vi "Reentrant SubVI.vi"(11 "Instance":i32) -> ()   [LabVIEW 2023]
doc: "This reentrant subVI is used by the Reentrant VI Execution.vi example. Based on the numeric input to the Instance control, a message is written to the string indicator notifying the user whether the first or second instance of the subVI has been called."
panel:
  in  "Message String":string="This is instance %d of the reentrant subVI."
  out "Message":string
  in  "Stop":bool
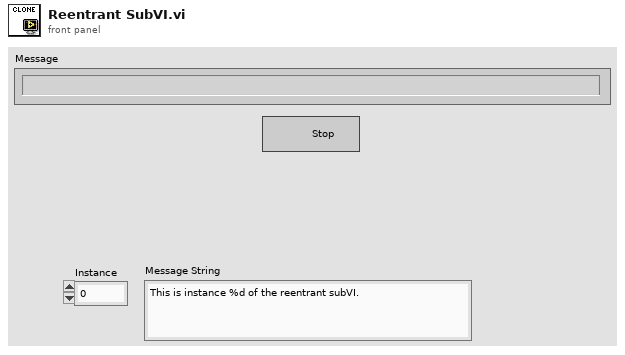
[diagram p1: front panel]
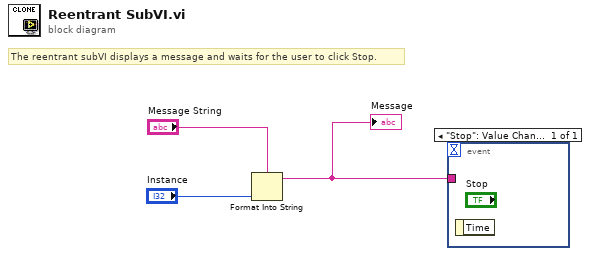
[diagram p0: block diagram]
diagram:
  # "The reentrant subVI displays a message and waits for the user to click Stop."
  n1 = Format Into String(format string="Message String", "Instance") -> (resulting string=w1:string)  [unwired: 2 in, 1 out]
  "Message" <- w1
  n2 = event shown="[0] \"Stop\": Value Change" {
    selector: _ -> [_]
    dyn-events: _ -> [_]
    timeout: _ -> [_]
    tunnel: w1 -> [_]
    event "Stop": Value Change {
      n3 = event-data() -> ()  [unwired: 1 in, 1 out]
    }
  }
